vi "Bind To Name.vi"(8 "error in (no error)":errorcluster, 10 "Type":refnum<class>, 11 "JSON Serializable Binder in":refnum<class "JSON Serializable Binder.lvclass">) -> (0 "error out":errorcluster, 2 "Type Name":string, 3 "JSON Serializable Binder out":refnum<class "JSON Serializable Binder.lvclass">)   [LabVIEW 2017, in "JSON Serializable Binder.lvclass"]
doc: "Controls the binding of a type to a serialized object."
uses:
  JSON Serializable Binder.lvclass
  JSON Serializable/JSON Serializable.lvclass
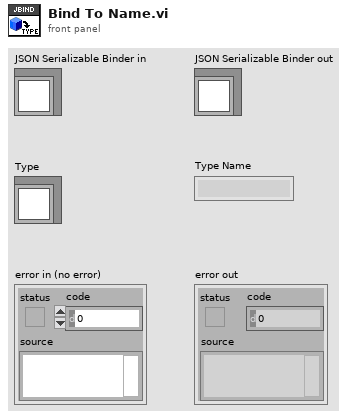
[diagram p1: front panel]
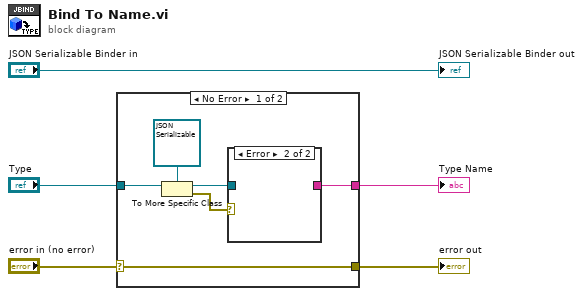
[diagram p0: block diagram]
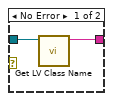
[diagram p2: hidden frame]
diagram:
  n1 = case shown="No Error" "error in (no error)" {
    selector: "error in (no error)" -> [w6 w14]
    tunnel: [w11 _] -> w4
    tunnel: "Type" -> [w9 _]
    tunnel: [w6 w14] -> w1
    frame No Error {
      n2 = To More Specific Class(target class=refnum<class "JSON Serializable.lvclass"> refnum ("JSON Serializable.lvclass"), reference=w9) -> (specific class reference=w8:refnum<class "JSON Serializable.lvclass">, error out=w7:errorcluster)  [unwired: 1 in]
      n3 = case shown="Error" w7 {
        tunnel: [w13 _] -> w11
        tunnel: w8 -> [w12 _]
        frame No Error {
          n4 = call <vilib>:"Get LV Class Name.vi"("object"=w12) -> ("class name"=w13:string)  [unwired: 9 in, 1 out]
        }
        frame Error {
        }
      }
    }
    frame Error {
    }
  }
  "error out" <- w1
  "Type Name" <- w4
  "JSON Serializable Binder out" <- "JSON Serializable Binder in"
